vi "Observe Data.vi"(6 "Time Stamp":timestamp, 8 "error in (no error)":errorcluster, 9 "Value":variant, 10 "Datum Name":string, 11 "DialogBoxSubscribesToDblX in":refnum<class "DialogBoxSubscribesToDblX.lvclass">) -> (0 "error out":errorcluster, 3 "DialogBoxSubscribesToDblX out":refnum<class "DialogBoxSubscribesToDblX.lvclass">)   [LabVIEW 2018, in "DialogBoxSubscribesToDblX.lvclass"]
doc: "<License>\nCopyright © 2017 Composed Systems, LLC | All rights reserved\nwww.composed.io\n\nAuthor: Ethan Stern <ethan.stern@composed.io>\n\nThis software is provided \"AS IS\" WITHOUT WARRANTIES, either express or implied, AND IS FOR EDUCATIONAL PURPOSES ONLY.\n</License>"
uses:
  DialogBoxSubscribesToDblX.lvclass
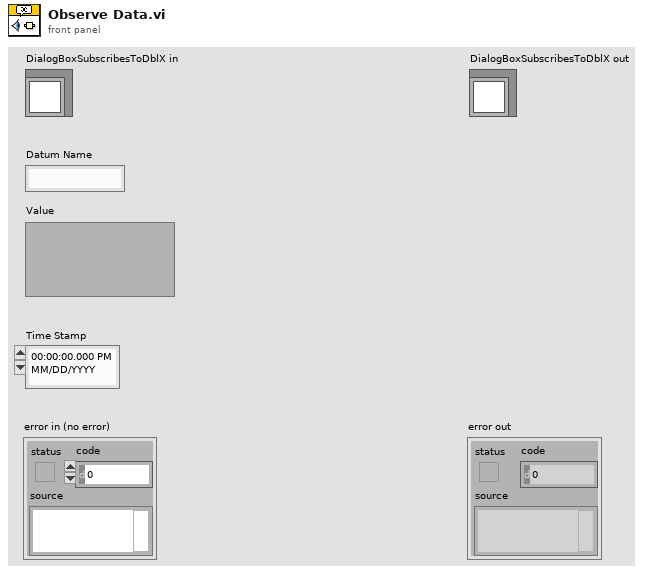
[diagram p1: front panel]
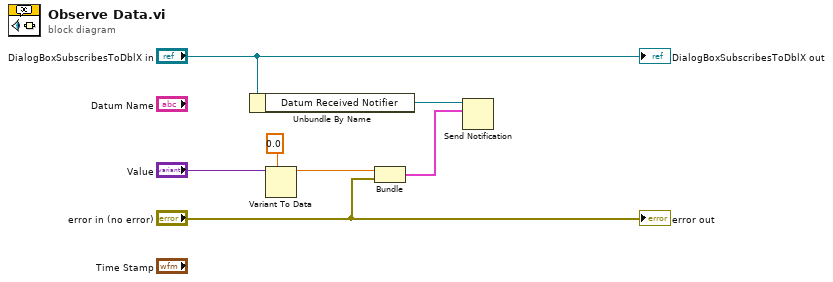
[diagram p0: block diagram]
diagram:
  n1 = Unbundle By Name("DialogBoxSubscribesToDblX in") -> ("Datum Received Notifier"=w6:refnum<notifier>)
  n2 = Variant To Data(type=0.0, Variant="Value") -> (data=w2:dbl)  [unwired: 1 in, 1 out]
  n3 = Bundle(w2, "error in (no error)"="error in (no error)") -> (w1:cluster{dbl, "error in (no error)":errorcluster})  [unwired: 1 in]
  n4 = Send Notification(notification=w1, notifier=w6) -> ()  [unwired: 1 in, 2 out]
  "error out" <- "error in (no error)"
  "DialogBoxSubscribesToDblX out" <- "DialogBoxSubscribesToDblX in"
